vi "Add-UpdateSailingPoints.vi"(7 "Has the first mission changed?":bool, 9 "NotifierReff":T1, 10 "Mission Notifiers":T2, 11 "Waypoints queue for Midbrain":refnum<queue>) -> (1 "Number of sailing points added":i32, 2 "Added sailing points?":bool, 3 "Added intermediate point?":bool)   [LabVIEW 2013]
uses:
  Classes/Waypoint/Waypoint.lvclass
  Data/TypeDefs/MissionNotifiers.ctl
  Classes/Missions/GenericMission/GenericMission.lvclass
  Classes/Obstacle/Obstacle.lvclass
  Data/TypeDefs/Notifiers.ctl
  Data/TypeDefs/UTM Location.ctl
  Data/TypeDefs/Sail Set Suggestions.ctl
  Data/TypeDefs/Rudder Set Suggestions.ctl
  Data/TypeDefs/OverrideInformation.ctl
  Data/TypeDefs/OverrideMode.ctl
  Data/TypeDefs/MotorSetup.ctl
  Data/TypeDefs/DynamixelSetupInfo.ctl
  Data/TypeDefs/AirmarStatus.ctl
  Data/TypeDefs/HardwareOnline.ctl
  Data/TypeDefs/DynamixelCycleTracker.ctl
  Data/TypeDefs/RC Input Values.ctl
  Utilities/Math/Angles/Angle/Angle.lvclass
panel:
  in  "Cutoff wind shift for recalc (deg) (10)":dbl=10.0
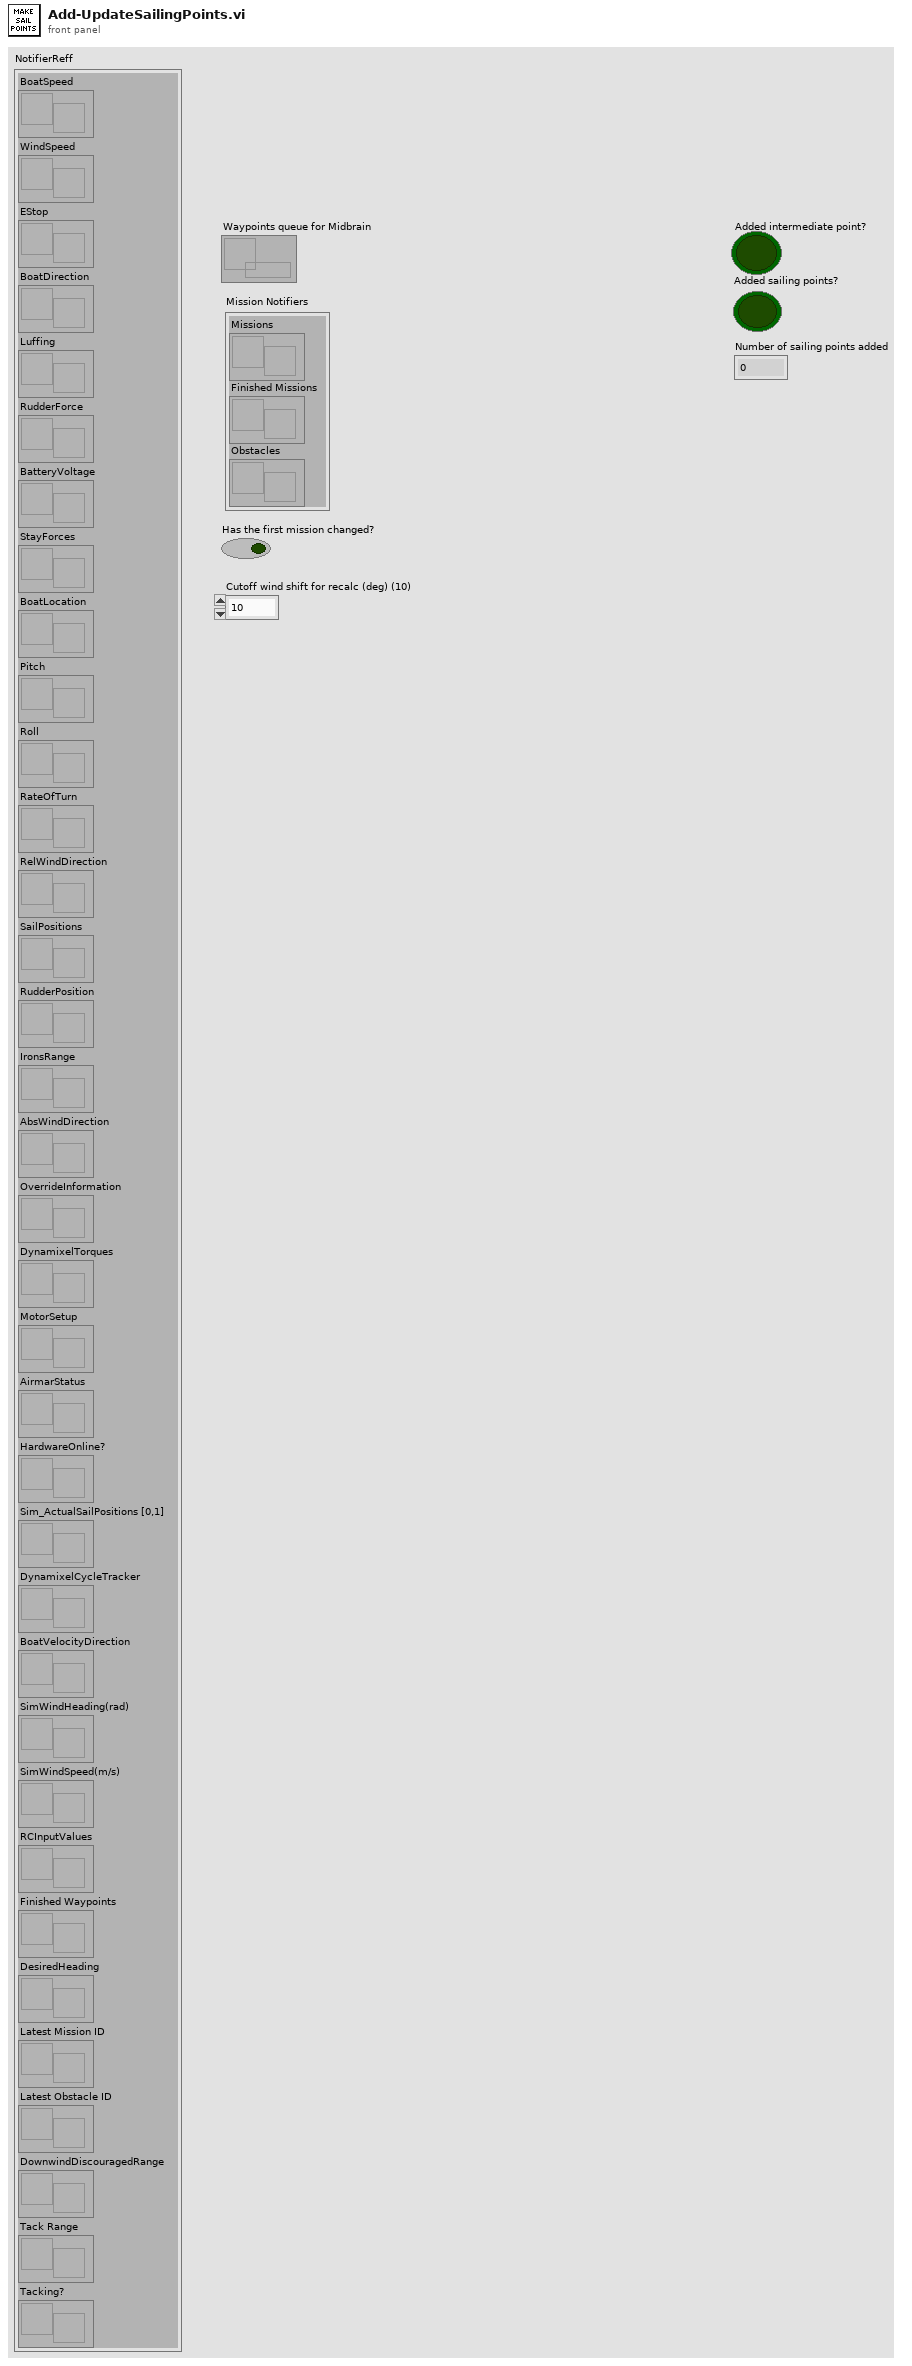
[diagram p1: front panel]
types:
  T1 = typedef "Notifiers.ctl" = cluster{"BoatSpeed":refnum<notifier>, "WindSpeed":refnum<notifier>, "EStop":refnum<notifier>, "BoatDirection":refnum<notifier>, "Luffing":refnum<notifier>, "RudderForce":refnum<notifier>, "BatteryVoltage":refnum<notifier>, "StayForces":refnum<notifier>, "BoatLocation":refnum<notifier>, "Pitch":refnum<notifier>, "Roll":refnum<notifier>, "RateOfTurn":refnum<notifier>, "RelWindDirection":refnum<notifier>, "SailPositions":refnum<notifier>, "RudderPosition":refnum<notifier>, "IronsRange":refnum<notifier>, "AbsWindDirection":refnum<notifier>, "OverrideInformation":refnum<notifier>, "DynamixelTorques":refnum<notifier>, "MotorSetup":refnum<notifier>, "AirmarStatus":refnum<notifier>, "HardwareOnline?":refnum<notifier>, "Sim_ActualSailPositions [0,1]":refnum<notifier>, "DynamixelCycleTracker":refnum<notifier>, "BoatVelocityDirection":refnum<notifier>, "SimWindHeading(rad)":refnum<notifier>, "SimWindSpeed(m/s)":refnum<notifier>, "RCInputValues":refnum<notifier>, "Finished Waypoints":refnum<notifier>, "DesiredHeading":refnum<notifier>, "Latest Mission ID":refnum<notifier>, "Latest Obstacle ID":refnum<notifier>, "DownwindDiscouragedRange":refnum<notifier>, "Tack Range":refnum<notifier>, "Tacking?":refnum<notifier>}
  T2 = typedef "MissionNotifiers.ctl" = cluster{"Missions":refnum<notifier>, "Finished Missions":refnum<notifier>, "Obstacles":refnum<notifier>}
  T3 = typedef "UTM Location.ctl" = cluster{"UTM Zone":dbl, "Hemisphere":enum16{"North", "South"}, "East":dbl, "North":dbl}
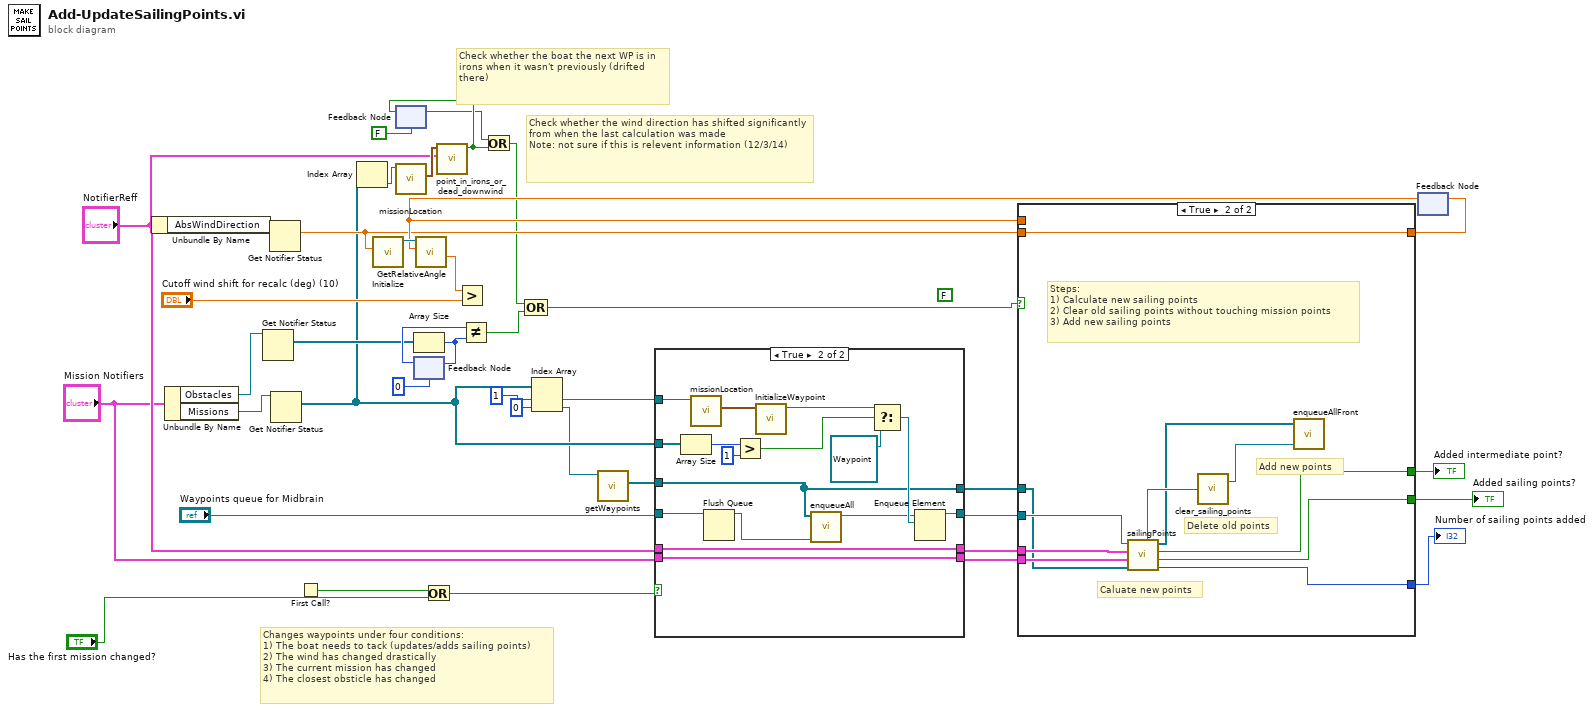
[diagram p0: block diagram]
diagram:
  (unwired) FALSE
  # "Changes waypoints under four conditions:\n1) The boat needs to tack (updates/adds sailing points)\n2) The wind has changed drastically\n3) The current mission has changed\n4) The closest obsticle has changed"
  # "Check whether the wind direction has shifted significantly from when the last calculation was made\nNote: not sure if this is relevent information (12/3/14)"
  # "Check whether the boat the next WP is in irons when it wasn't previously (drifted there)"
  n1 = Unbundle By Name("NotifierReff") -> ("AbsWindDirection"=w40:refnum<notifier>)
  n2 = Unbundle By Name("Mission Notifiers") -> ("Obstacles"=w24:refnum<notifier>, "Missions"=w25:refnum<notifier>)
  n3 = Get Notifier Status(notifier=w24) -> (current notification=w28:refnum<class "Obstacle.lvclass">[])  [unwired: 1 in, 4 out]
  n4 = Get Notifier Status(notifier=w40) -> (current notification=w34:dbl)  [unwired: 1 in, 4 out]
  n5 = Get Notifier Status(notifier=w25) -> (current notification=w10:refnum<class "GenericMission.lvclass">[])  [unwired: 1 in, 4 out]
  n6 = First Call?() -> (First Call?: T/F=w3:bool)
  n7 = Index Array(array=w10) -> (element=w27:refnum<class "GenericMission.lvclass">)  [unwired: 1 in]
  n8 = call "Initialize.vi"("Input Angle (Deg.)"=w34) -> ("Angle out"=w37:refnum<class "Angle.lvclass">)  [unwired: 9 in, 1 out]
  n9 = feedback #1(FALSE ("In irons or dead downwind?")) -> (w30:bool)
  n10 = call-dynamic "missionLocation.vi"("GenericMission in"=w27) -> ("element"=w26:T3)  [unwired: 8 in, 2 out]
  n11 = Array Size(array=w28) -> (size(s)=w38:i32)
  n12 = feedback-in #2(w38) -> ()
  n13 = feedback #2(0) -> (w39:i32)
  n14 = Or(x=w3, y="Has the first mission changed?") -> (x .or. y?=w1:bool)
  n15 = call "point_in_irons_or_dead_downwind.vi"("NotifierReff"="NotifierReff", "Point"=w26) -> ("In irons or dead downwind?"=w31:bool)  [unwired: 7 in, 2 out]
  n16 = feedback-in #1(w31) -> ()
  n17 = Not Equal?(x=w39, y=w38) -> (x != y?=w17:bool)
  n18 = Or(x=w30, y=w31) -> (x .or. y?=w29:bool)
  n19 = Compound Arithmetic op=OR(w29, w17) -> (w4:bool)
  n20 = Index Array(array=w10, index #1=1 ("index"), index #2=0 ("index")) -> (element #1=w8:refnum<class "GenericMission.lvclass">, element #2=w7:refnum<class "GenericMission.lvclass">)
  n21 = call-dynamic "getWaypoints.vi"("GenericMission in"=w7) -> ("Waypoint Array"=w6:refnum<class "Waypoint.lvclass">[])  [unwired: 8 in, 2 out]
  n22 = case shown="True" w1 {
    tunnel: "Waypoints queue for Midbrain" -> [w44 w58]
    tunnel: [w43 w60] -> w14
    tunnel: "NotifierReff" -> [w43 w60]
    tunnel: [w42 w59] -> w13
    tunnel: "Mission Notifiers" -> [w42 w59]
    tunnel: w8 -> [_ w54]
    tunnel: w10 -> [_ w57]
    tunnel: [w44 w49] -> w9
    tunnel: w6 -> [w41 w45]
    tunnel: [w41 w45] -> w5
    frame False {
    }
    frame True {
      n23 = Array Size(array=w57) -> (size(s)=w56:i32)
      n24 = call-dynamic "missionLocation.vi"("GenericMission in"=w54) -> ("element"=w53:T3)  [unwired: 8 in, 2 out]
      n25 = Flush Queue(queue=w58) -> (queue out=w47:refnum<queue>)  [unwired: 1 in, 2 out]
      n26 = Greater?(x=w56, y=1) -> (0:w52:bool)
      n27 = call "InitializeWaypoint.vi"("Coords"=w53) -> ("Waypoint Out"=w51:refnum<class "Waypoint.lvclass">)  [unwired: 10 in]
      n28 = call "enqueueAll.vi"("Waypoint Queue"=w47, "Waypoint Array"=w45) -> ("Waypoint Queue Out"=w46:refnum<queue>)  [unwired: 9 in]
      n29 = Select(t=w51, s=w52, f=refnum<class "Waypoint.lvclass"> refnum ("Waypoint.lvclass")) -> (s? t:f=w48:refnum<class "Waypoint.lvclass">)
      n30 = Enqueue Element(queue=w46, element=w48) -> (queue out=w49:refnum<queue>)  [unwired: 2 in, 2 out]
    }
  }
  n31 = feedback #3() -> (w35:dbl)  [unwired: 1 in]
  n32 = call "GetRelativeAngle.vi"("Boat Heading (Deg.)"=w35, "Angle in"=w37) -> ("Absolute difference (deg)"=w32:dbl)  [unwired: 6 in, 3 out]
  n33 = Greater?(x=w32, y="Cutoff wind shift for recalc (deg) (10)") -> ()  [unwired: 1 out]
  n34 = case shown="True" w4 {
    tunnel: [w61 w72] -> w36
    tunnel: w35 -> [w61 _]
    tunnel: w34 -> [_ w72]
    tunnel: w14 -> [_ w68]
    tunnel: w13 -> [_ w67]
    tunnel: [_ w71] -> w21
    tunnel: [_ w70] -> w20
    tunnel: [_ w69] -> w19
    tunnel: w9 -> [_ w65]
    tunnel: w5 -> [_ w64]
    frame False {
    }
    frame True {
      # "Add new points"
      # "Delete old points"
      # "Caluate new points"
      # "Steps:\n1) Calculate new sailing points\n2) Clear old sailing points without touching mission points\n3) Add new sailing points"
      n35 = call "sailingPoints.vi"("Waypoint Array"=w64, "Mission Notifiers"=w67, "NotifierReff"=w68, "Waypoint queue"=w65) -> ("Number of sailing points added"=w69:i32, "Added sailing points?"=w70:bool, "Added intermediate point?"=w71:bool, "New Sailing points"=w63:refnum<class "Waypoint.lvclass">[], "Waypoint queue out"=w66:refnum<queue>)  [unwired: 3 in]
      n36 = call "clear_sailing_points.vi"("Waypoints queue"=w66) -> ("Waypoints queue 2"=w62:refnum<queue>)  [unwired: 1 out]
      n37 = call "enqueueAllFront.vi"("Waypoint Queue"=w62, "Waypoint Array"=w63) -> ()  [unwired: 1 in, 1 out]
    }
  }
  "Added intermediate point?" <- w21
  "Added sailing points?" <- w20
  "Number of sailing points added" <- w19
  n38 = feedback-in #3(w36) -> ()
